vi "MB ICPCON Registers Manager Init.vi"(8 "error in (no error)":errorcluster, 11 "Data Buffer Length":i32=1000) -> (0 "error out":errorcluster, 3 "Data Reference":T1)   [LabVIEW 2019, in "ICPCON Registers.lvlib"]
uses:
  ICPCON Registers.lvlib
  Ctl/ICPCON Data.ctl
  Timer Delay/unix time 1ms.vi
  Timer Delay/Timers.lvlib
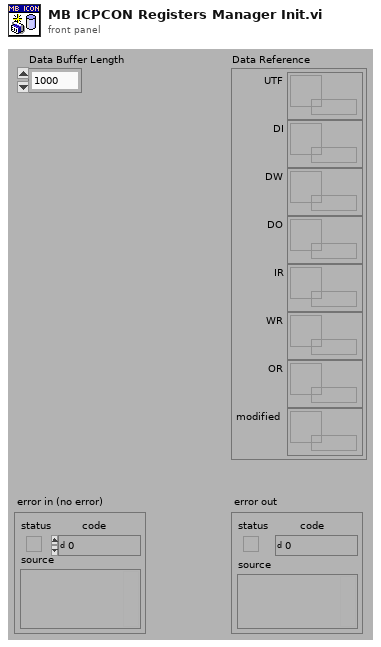
[diagram p1: front panel]
types:
  T1 = typedef "ICPCON Registers.lvlib/ICPCON Data.ctl" = cluster{"UTF":refnum<data-value>, "DI":refnum<data-value>, "DW":refnum<data-value>, "DO":refnum<data-value>, "IR":refnum<data-value>, "WR":refnum<data-value>, "OR":refnum<data-value>, "modified":refnum<data-value>}
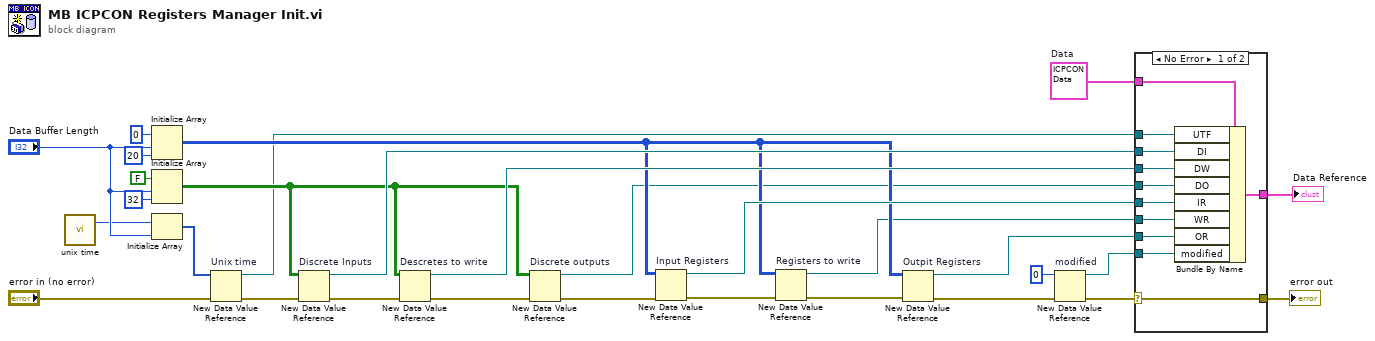
[diagram p0: block diagram]
diagram:
  w25 = T1 {"UTF"=refnum, "DI"=refnum, "DW"=refnum, "DO"=refnum, "IR"=refnum, "WR"=refnum, "OR"=refnum, "modified"=refnum}  # Data
  n1 = call-poly "unix time.vi"() -> ("unix time (ms)"=w7:u64)  [unwired: 2 in, 1 out]
  n2 = Initialize Array(u16 0, "Data Buffer Length", 20 ("dimension size")) -> (w13:u16[][])
  n3 = Initialize Array(FALSE, "Data Buffer Length", 32 ("dimension size")) -> (w18:bool[][])
  n4 = Initialize Array(w7, "Data Buffer Length") -> (w8:u64[])
  n5 = New Data Value Reference "Unix time"(data value=w8) -> (data value reference=w6:refnum<data-value>)  [unwired: 1 in, 1 out]
  n6 = New Data Value Reference "Discrete Inputs"(data value=w18, error in="error in (no error)") -> (data value reference=w24:refnum<data-value>, error out=w26:errorcluster)
  n7 = New Data Value Reference "Descretes to write"(data value=w18, error in=w26) -> (data value reference=w23:refnum<data-value>, error out=w19:errorcluster)
  n8 = New Data Value Reference "Discrete outputs"(data value=w18, error in=w19) -> (data value reference=w12:refnum<data-value>, error out=w20:errorcluster)
  n9 = New Data Value Reference "Input Registers"(data value=w13, error in=w20) -> (data value reference=w22:refnum<data-value>, error out=w15:errorcluster)
  n10 = New Data Value Reference "Registers to write"(data value=w13, error in=w15) -> (data value reference=w11:refnum<data-value>, error out=w14:errorcluster)
  n11 = New Data Value Reference "Outpit Registers"(data value=w13, error in=w14) -> (data value reference=w21:refnum<data-value>, error out=w3:errorcluster)
  n12 = New Data Value Reference "modified"(data value=u8 0 ("modified"), error in=w3) -> (data value reference=w4:refnum<data-value>, error out=w2:errorcluster)
  n13 = case shown="No Error" w2 {
    selector: w2 -> [w30 w42]
    tunnel: w25 -> [w40 w41]
    tunnel: w24 -> [w39 _]
    tunnel: w23 -> [w38 _]
    tunnel: w22 -> [w37 _]
    tunnel: w21 -> [w36 _]
    tunnel: w12 -> [w35 _]
    tunnel: w11 -> [w34 _]
    tunnel: [w33 w41] -> w10
    tunnel: w6 -> [w32 _]
    tunnel: w4 -> [w31 _]
    tunnel: [w30 w42] -> w1
    frame No Error {
      n14 = Bundle By Name(cluster=w40, "UTF"=w32, "DI"=w39, "DW"=w38, "DO"=w35, "IR"=w37, "WR"=w34, "OR"=w36, "modified"=w31) -> (w33:T1)
    }
    frame Error {
    }
  }
  "error out" <- w1
  "Data Reference" <- w10
